vi "Chamber Response Simulator AE.vi"(7 "Thermal Chamber Function":T1, 8 "error in (no error)":errorcluster, 9 "Time Interval (ms)":u32, 10 "Ramp Rate in":dbl, 11 "Temperature Set Point in":dbl) -> (0 "error out":errorcluster, 2 "Ramp Rate out":dbl, 3 "Temperature Set Point out":dbl, 4 "Application Exit":bool, 5 "Actual Temperature":dbl, 6 "Shutdown Furnace?":bool)   [LabVIEW 2015, in "Thermal Chamber Response Simulator.lvlib"]
doc: "The action engine that provides the simulated response of the temperature chamber.\n____\nDelacor QMH Thermal Chamber Examples 4.0.0.21\nCopyright (c) 2018, Delacor"
uses:
  Thermal Chamber Response Simulator.lvlib
  Action--enum.ctl
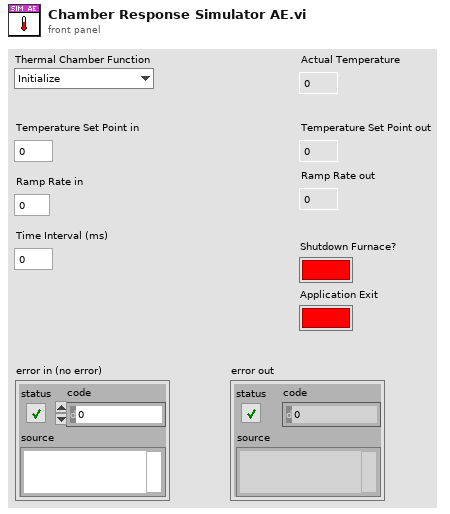
[diagram p1: front panel]
types:
  T1 = typedef "Thermal Chamber Response Simulator.lvlib/Action--enum.ctl" = enum16{"Initialize", "Set Temperature Required", "Set Ramp Rate", "Get Status", "Disable Heater", "Enable Heater", "Exit Application"}
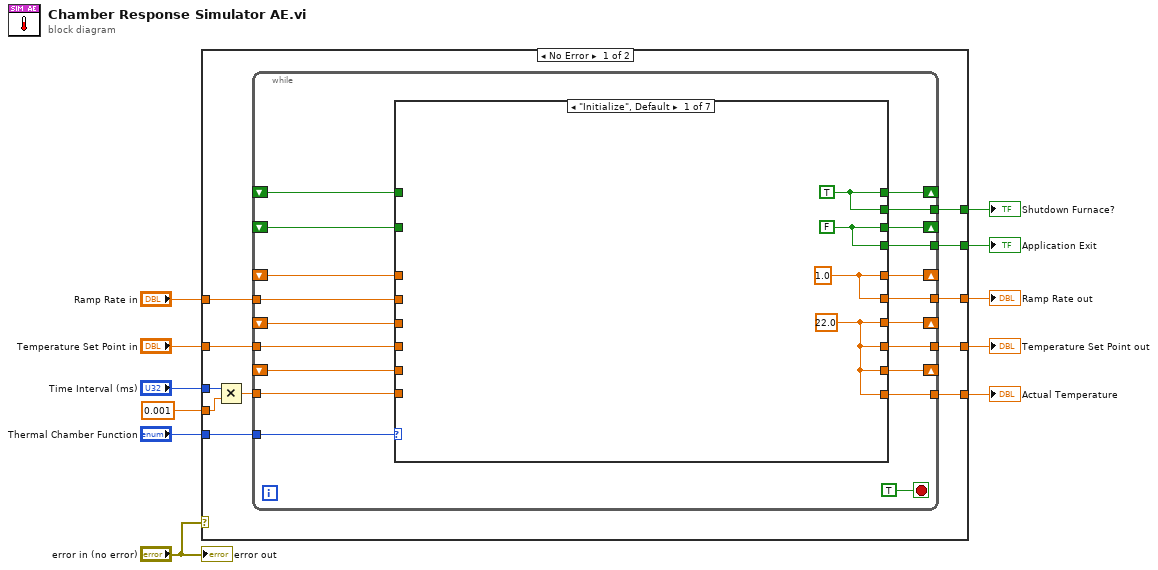
[diagram p0: block diagram]
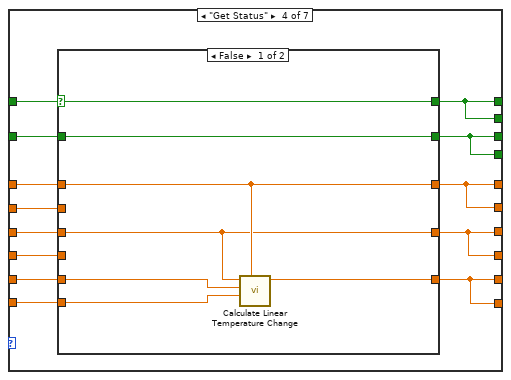
[diagram p4: hidden frame]
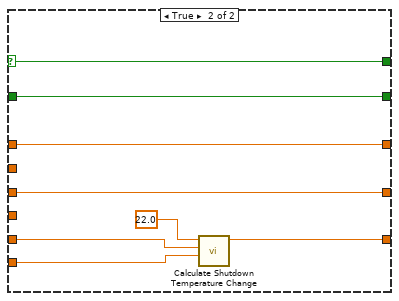
[diagram p5: hidden frame]
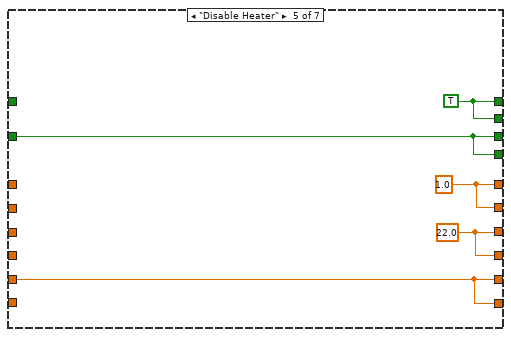
[diagram p6: hidden frame]
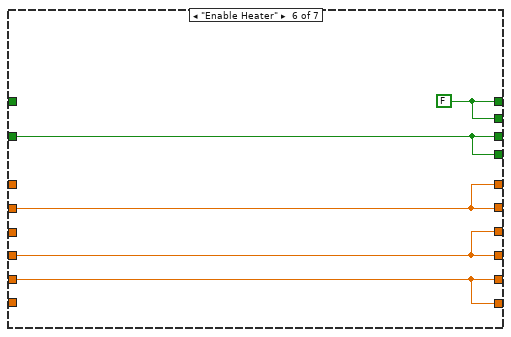
[diagram p7: hidden frame]
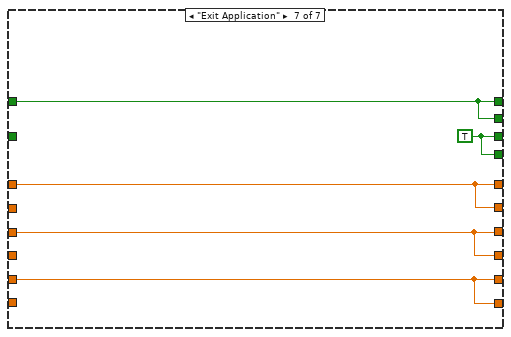
[diagram p8: hidden frame]
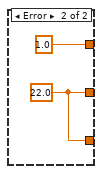
[diagram p9: hidden frame]
diagram:
  n1 = case shown="No Error" "error in (no error)" {
    tunnel: "Thermal Chamber Function" -> [w22 _]
    tunnel: "Temperature Set Point in" -> [w21 _]
    tunnel: "Ramp Rate in" -> [w20 _]
    tunnel: "Time Interval (ms)" -> [w19 _]
    tunnel: 0.001 ("y") -> [w18 _]
    tunnel: [w16 _] -> w6
    tunnel: [w15 _] -> w5
    tunnel: [w14 1.0] -> w4
    tunnel: [w13 w100] -> w3
    tunnel: [w12 w100] -> w2
    frame No Error {
      n2 = Multiply(x=w19, y=w18) -> (x*y=w17:dbl)
      n3 = while {
        tunnel: w22 -> [w23]
        tunnel: w21 -> [w42]
        tunnel: w20 -> [w41]
        tunnel: w17 -> [w40]
        shift-right: [w32] -> _
        shift-left: _ -> [w26]
        shift-right: [w30] -> _
        shift-left: _ -> [w25]
        shift-right: [w28] -> _
        shift-left: _ -> [w24]
        shift-right: [w38] -> _
        shift-left: _ -> [w34]
        shift-right: [w37] -> _
        shift-left: _ -> [w33]
        tunnel: [w36] -> w15
        tunnel: [w35] -> w16
        tunnel: [w31] -> w14
        tunnel: [w29] -> w13
        tunnel: [w27] -> w12
        stop <- TRUE stop-if-true
        n4 = case shown="\"Initialize\", Default" w23 {
          tunnel: w42 -> [_ w48 _ w65 _ w93 _]
          tunnel: w41 -> [_ _ w54 w67 _ w92 _]
          tunnel: w40 -> [_ _ _ w63 _ _ _]
          tunnel: [w46 w51 w56 w59 w88 w91 w99] -> w38
          tunnel: [w45 w50 w55 w57 w89 w90 w95] -> w37
          tunnel: [w46 w51 w56 w59 w88 w91 w99] -> w36
          tunnel: [w45 w50 w55 w57 w89 w90 w95] -> w35
          tunnel: w34 -> [_ w51 w56 w69 _ _ w99]
          tunnel: w33 -> [_ w50 w55 w58 w89 w90 _]
          tunnel: [w44 w49 w54 w62 w85 w92 w98] -> w32
          tunnel: [w44 w49 w54 w62 w85 w92 w98] -> w31
          tunnel: [w43 w48 w53 w61 w86 w93 w97] -> w30
          tunnel: [w43 w48 w53 w61 w86 w93 w97] -> w29
          tunnel: [w43 w47 w52 w60 w87 w94 w96] -> w28
          tunnel: [w43 w47 w52 w60 w87 w94 w96] -> w27
          tunnel: w26 -> [_ w49 _ w68 _ _ w98]
          tunnel: w25 -> [_ _ w53 w66 _ _ w97]
          tunnel: w24 -> [_ w47 w52 w64 w87 w94 w96]
          frame "Initialize", Default {
            w43 = 22.0
            w44 = 1.0
            w45 = FALSE
            w46 = TRUE
          }
          frame "Set Temperature Required" {
          }
          frame "Set Ramp Rate" {
          }
          frame "Get Status" {
            n5 = case shown="False" w69 {
              selector: w69 -> [w70 w80]
              tunnel: w68 -> [w76 w81]
              tunnel: w67 -> [_ _]
              tunnel: w66 -> [w75 w83]
              tunnel: w65 -> [_ _]
              tunnel: w64 -> [w74 w78]
              tunnel: w63 -> [w73 w82]
              tunnel: [w76 w81] -> w62
              tunnel: [w75 w83] -> w61
              tunnel: [w72 w84] -> w60
              tunnel: [w70 w80] -> w59
              tunnel: w58 -> [w71 w79]
              tunnel: [w71 w79] -> w57
              frame False {
                n6 = call "Calculate Linear Temperature Change.vi"("Ramp Rate deg C/s"=w76, "Time Interval (s)"=w73, "Actual Temperature in"=w74, "Required Temperature deg C"=w75) -> ("Actual Temperature out"=w72:dbl)  [unwired: 7 in]
              }
              frame True {
                n7 = call "Calculate Shutdown Temperature Change.vi"("Interval"=w82, "Actual Temperature In"=w78, "Required Temperature deg C"=22.0) -> ("Actual Temperature Out"=w84:dbl)  [unwired: 8 in]
              }
            }
          }
          frame "Disable Heater" {
            w85 = 1.0
            w86 = 22.0
            w88 = TRUE
          }
          frame "Enable Heater" {
            w91 = FALSE
          }
          frame "Exit Application" {
            w95 = TRUE
          }
        }
      }
    }
    frame Error {
      w100 = 22.0
    }
  }
  "Actual Temperature" <- w2
  "Temperature Set Point out" <- w3
  "Ramp Rate out" <- w4
  "Shutdown Furnace?" <- w5
  "Application Exit" <- w6
  "error out" <- "error in (no error)"
